vi "testCamera.vi"() -> ()   [LabVIEW 2011, in "run.lvlib"]
uses:
  run.lvlib
  Tools/CameraSettings/CamaraSettings.lvclass
  Channels/Camera/Camera/Camera.lvclass
panel:
  in  "savePath":path
  in  "cameraSetting":path
  in  "number":i32=-1
  out "stopped":bool
  out "imageSaved":bool
  out "temperature":dbl
  in  "stop":bool
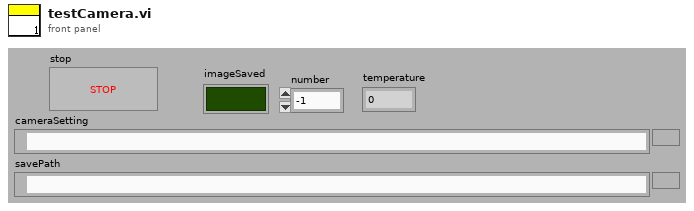
[diagram p1: front panel]
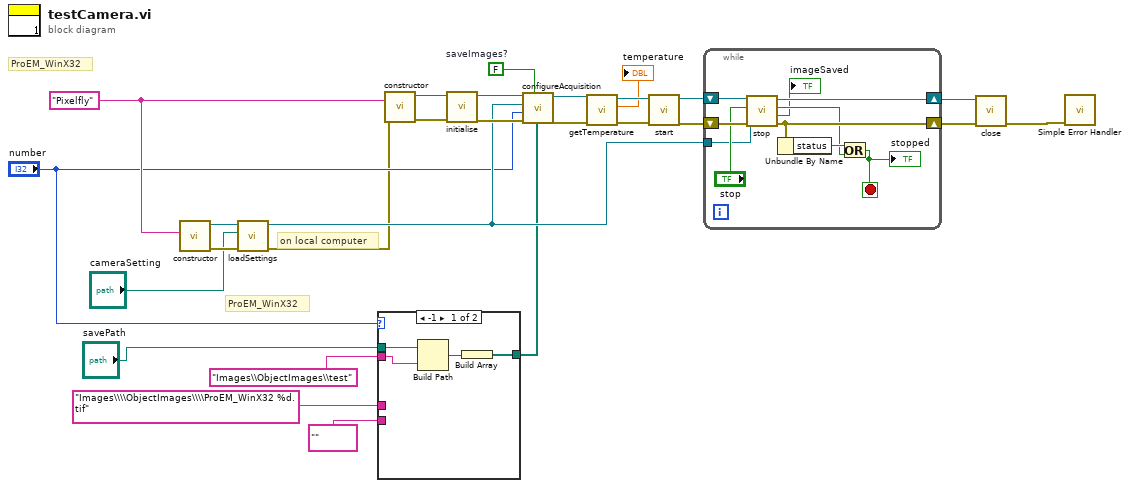
[diagram p0: block diagram]
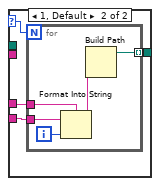
[diagram p2: hidden frame]
diagram:
  w12 = FALSE  # saveImages?
  w18 = "Pixelfly" ("Camera")
  # "ProEM_WinX32"
  # "ProEM_WinX32"
  # "on local computer"
  n1 = call "constructor.vi"("camera settings"=w18) -> ("error out"=w16:errorcluster, "CamaraSettings out"=w17:refnum<class "CamaraSettings.lvclass">)  [unwired: 9 in]
  n2 = call-dynamic "loadSettings.vi"("error in (no error)"=w16, "Path"="cameraSetting", "CamaraSettings in"=w17) -> ("error out"=w2:errorcluster, "CamaraSettings out"=w15:refnum<class "CamaraSettings.lvclass">)  [unwired: 7 in]
  n3 = case shown="-1" "number" {
    selector: "number" -> [_ w33]
    tunnel: [w31 w35] -> w4
    tunnel: "Images\\\\ObjectImages\\\\ProEM_WinX32 %d.tif" -> [_ w34]
    tunnel: "" -> [_ w32]
    tunnel: "Images\\ObjectImages\\test" -> [w30 _]
    tunnel: "savePath" -> [w28 _]
    frame -1 {
      n4 = Build Path(base path=w28, name or relative path=w30) -> (appended path=w29:path)
      n5 = Build Array(w29) -> (w31:path[])
    }
    frame 1, Default {
      n6 = for {
        N: w33 -> [_]
        tunnel: [w40] -> w35 mode=indexing
        tunnel: w34 -> [w38]
        tunnel: w32 -> [w36]
        i -> [w39]
        n7 = Format Into String(format string=w38, initial string=w36, w39) -> (resulting string=w37:string)  [unwired: 1 in, 1 out]
        n8 = Build Path(name or relative path=w37) -> (appended path=w40:path)  [unwired: 1 in]
      }
    }
  }
  n9 = call "constructor.vi"("error in (no error)"=w2, "Camera"=w18) -> ("error out"=w19:errorcluster, "Camera out"=w27:refnum<class "Camera.lvclass">)  [unwired: 8 in]
  n10 = call-dynamic "initialise.vi"("error in (no error)"=w19, "Camera in"=w27) -> ("error out"=w20:errorcluster, "Camera out"=w26:refnum<class "Camera.lvclass">)  [unwired: 8 in]
  n11 = call-dynamic "configureAcquisition.vi"("imagePaths"=w4, "saveImages?"=w12, "error in (no error)"=w20, "number of Images"="number", "CameraSettings"=w15, "Camera in"=w26) -> ("error out"=w21:errorcluster, "Camera out"=w25:refnum<class "Camera.lvclass">)  [unwired: 4 in]
  n12 = call-dynamic "getTemperature.vi"("error in (no error)"=w21, "Camera in"=w25) -> ("error out"=w10:errorcluster, "temperature"=→"temperature":dbl, "Camera out"=w24:refnum<class "Camera.lvclass">)  [unwired: 7 in]
  n13 = call-dynamic "start.vi"("error in (no error)"=w10, "Camera in"=w24) -> ("error out"=w22:errorcluster, "Camera out"=w23:refnum<class "Camera.lvclass">)  [unwired: 8 in]
  n14 = while {
    tunnel: w15 -> [w46]
    shift-right: [w49] -> w11
    shift-left: w23 -> [w50]
    shift-right: [w45] -> w13
    shift-left: w22 -> [w48]
    stop <- w42 stop-if-true
    n15 = call-dynamic "stop.vi"("error in (no error)"=w48, "CameraSettings"=w46, "stop"="stop", "Camera in"=w50) -> ("error out"=w45:errorcluster, "imageSaved"=→"imageSaved":bool, "stopped?"=w43:bool, "Camera out"=w49:refnum<class "Camera.lvclass">)  [unwired: 4 in]
    n16 = Unbundle By Name(w45) -> ("status"=w44:bool)
    n17 = Or(x=w44, y=w43) -> (x .or. y?=w42:bool)
    "stopped" <- w42
  }
  n18 = call-dynamic "close.vi"("error in (no error)"=w13, "Camera in"=w11) -> ("error out"=w9:errorcluster)  [unwired: 9 in]
  n19 = call <vilib>:"Simple Error Handler.vi"("error in (no error)"=w9) -> ()  [unwired: 4 in, 5 out]
